vi "Read Timestamp Options.vi"(11 "Serializer.JSON in":refnum<class "Serializer.JSON.lvclass">) -> (2 "Timestamp Serialization":T1, 3 "Serializer.JSON out":refnum<class "Serializer.JSON.lvclass">)   [LabVIEW 2013, in "OpenSerializer.JKI-JSON.lvlib" / "Serializer.JSON.lvclass"]
uses:
  Serializer.JSON.lvclass
  <vilib>/addons/_JKI.lib/Serialization/JSON/Library/Timestamp Options.ctl
  Serializer.JSON.lvclass/Serializer.JSON.ctl
  <vilib>/addons/_JKI.lib/Serialization/JSON/JKI JSON Serialization.lvlib
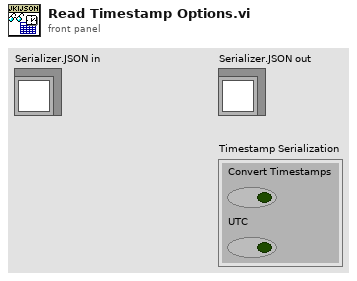
[diagram p1: front panel]
types:
  T1 = typedef "JKI JSON Serialization.lvlib/Timestamp Options.ctl" = cluster{"Convert Timestamps":bool, "UTC":bool}
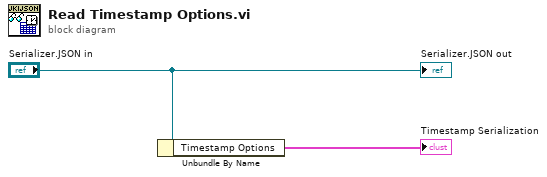
[diagram p0: block diagram]
diagram:
  n1 = Unbundle By Name("Serializer.JSON in") -> ("Timestamp Options"=→"Timestamp Serialization":T1)
  "Serializer.JSON out" <- "Serializer.JSON in"
